vi "S2C_VLFT10_Proc_VarStorageFGV.vi"(7 "Action":enum16{"Read", "Write", "Clear"}(ring), 8 "Error In":errorcluster, 11 "Data In":string[](array[string])) -> (0 "Error Out":errorcluster, 3 "Data Out":string[][](array[string]))   [LabVIEW 2015]
doc: "Detects an error and calls the error case to process the error."
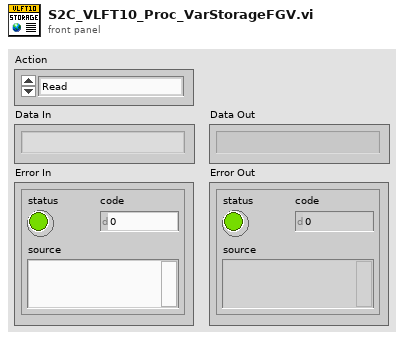
[diagram p1: front panel]
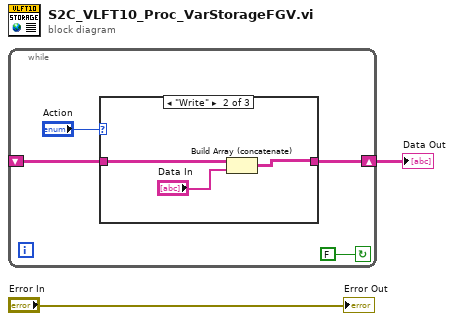
[diagram p0: block diagram]
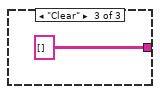
[diagram p3: hidden frame]
diagram:
  n1 = while {
    shift-right: [w4] -> w1
    shift-left: _ -> [w3]
    stop <- FALSE continue-if-true
    n2 = case shown="\"Write\"" "Action" {
      tunnel: [w7 w8 string[][] []] -> w4
      tunnel: w3 -> [w7 w10 _]
      frame "Read", Default {
      }
      frame "Write" {
        n3 = Build Array (concatenate)(w10, "Data In") -> (w8:string[][])
      }
      frame "Clear" {
      }
    }
  }
  "Data Out" <- w1
  "Error Out" <- "Error In"
